vi "删除数组空白.vi"(11 "all rows输入":string[](array[string])) -> (3 "all rows输出":string[](array[string]))   [LabVIEW 2017]
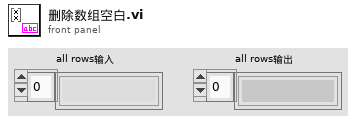
[diagram p1: front panel]
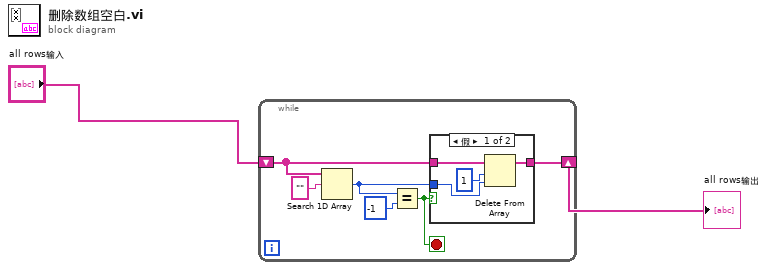
[diagram p0: block diagram]
diagram:
  n1 = while {
    shift-right: [w4] -> w2
    shift-left: "all rows输入" -> [w6]
    stop <- w5 stop-if-true
    n2 = Search 1D Array(1D array=w6, element="" ("元素")) -> (index of element=w3:i32)  [unwired: 1 in]
    n3 = Equal?(x=w3, y=-1) -> (x = y?=w5:bool)
    n4 = case shown="假" w5 {
      tunnel: w6 -> [w12 w13]
      tunnel: [w11 w13] -> w4
      tunnel: w3 -> [w10 _]
      frame False {
        n5 = Delete From Array(array=w12, length=1 ("长度"), index=w10) -> (array with subset deleted=w11:string[])  [unwired: 1 out]
      }
      frame True {
      }
    }
  }
  "all rows输出" <- w2
